vi "探头模板-12.vi"() -> ()   [LabVIEW 2017]
uses:
  <vilib>/Utility/miscctls.llb/LVPoint32TypeDef.ctl
  <vilib>/Utility/miscctls.llb/LVPositionTypeDef.ctl
panel:
  in  "鼠标坐标":T1 caption="坐标"
  out "计算时间":dbl
  in  "坐标映射信号":bool=TRUE
  in  "停止":bool=TRUE
  out "探头地址":T2(ring)
  out "探头状态":T3(ring)=enum."离线"
  out "探头信息":string
  out "测量值":dbl format="%.2g"
  out "单位":enum16{"μ", "m"}(ring)
  out "限值1":string="一级限值："
  out "限值2":string="二级限值："
  out "累积剂量":string="二级限值："
  in  "数据簇":T4
  out "数值":string
  in  "XY图":cluster{timestamp[], dbl[]}[](graph)
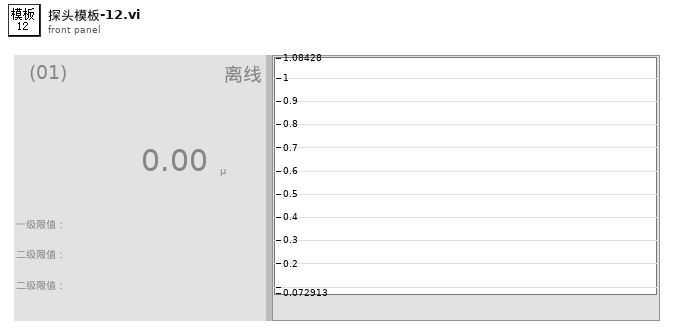
[diagram p1: front panel]
types:
  T1 = typedef "LVPoint32TypeDef.ctl" = cluster{"Horizontal":i32, "Vertical":i32}
  T2 = enum16{"(01)", "(02)", "(03)", "(04)", "(05)", "(06)", "(07)", "(08)", "(09)", "(10)", "(11)", "(12)", "(13)", "(14)", "(15)", "(16)", "(17)", "(18)", "(19)", "(20)", "(21)", "(22)", "(23)", "(24)", "(25)", "(26)", "(27)", "(28)", "(29)", "(30)", "(31)", "(32)", "(33)", "(34)", "(35)"}
  T3 = enum16{"正常", "未启用", "离线", "一级报警", "二级报警", "累积报警"}
  T4 = cluster{"启用状态？":bool, "测量值":cluster{"X":timestamp, "Y":dbl}, "限值簇":cluster{"限值1":dbl, "限值2":dbl, "探头限值":enum16{"一级限值", "二级限值"}}, "报警状态":enum16{"正常", "一级报警", "二级报警", "累积报警"}, "探头信息":string, "探头地址":i32, "累积剂量":cluster{"设备名称":string, "启用累积？":bool, "起始时间":timestamp, "累积剂量":dbl, "累积报警阈值":dbl}}
  T5 = typedef "LVPositionTypeDef.ctl" = cluster{"Left":i32, "Top":i32}
  T6 = cluster{"限值1":dbl, "限值2":dbl, "探头限值":enum16{"一级限值", "二级限值"}}
  T7 = cluster{"设备名称":string, "启用累积？":bool, "起始时间":timestamp, "累积剂量":dbl, "累积报警阈值":dbl}
  T8 = typedef "LVBoundsTypeDef.ctl" = cluster{"Width":u32, "Height":u32}
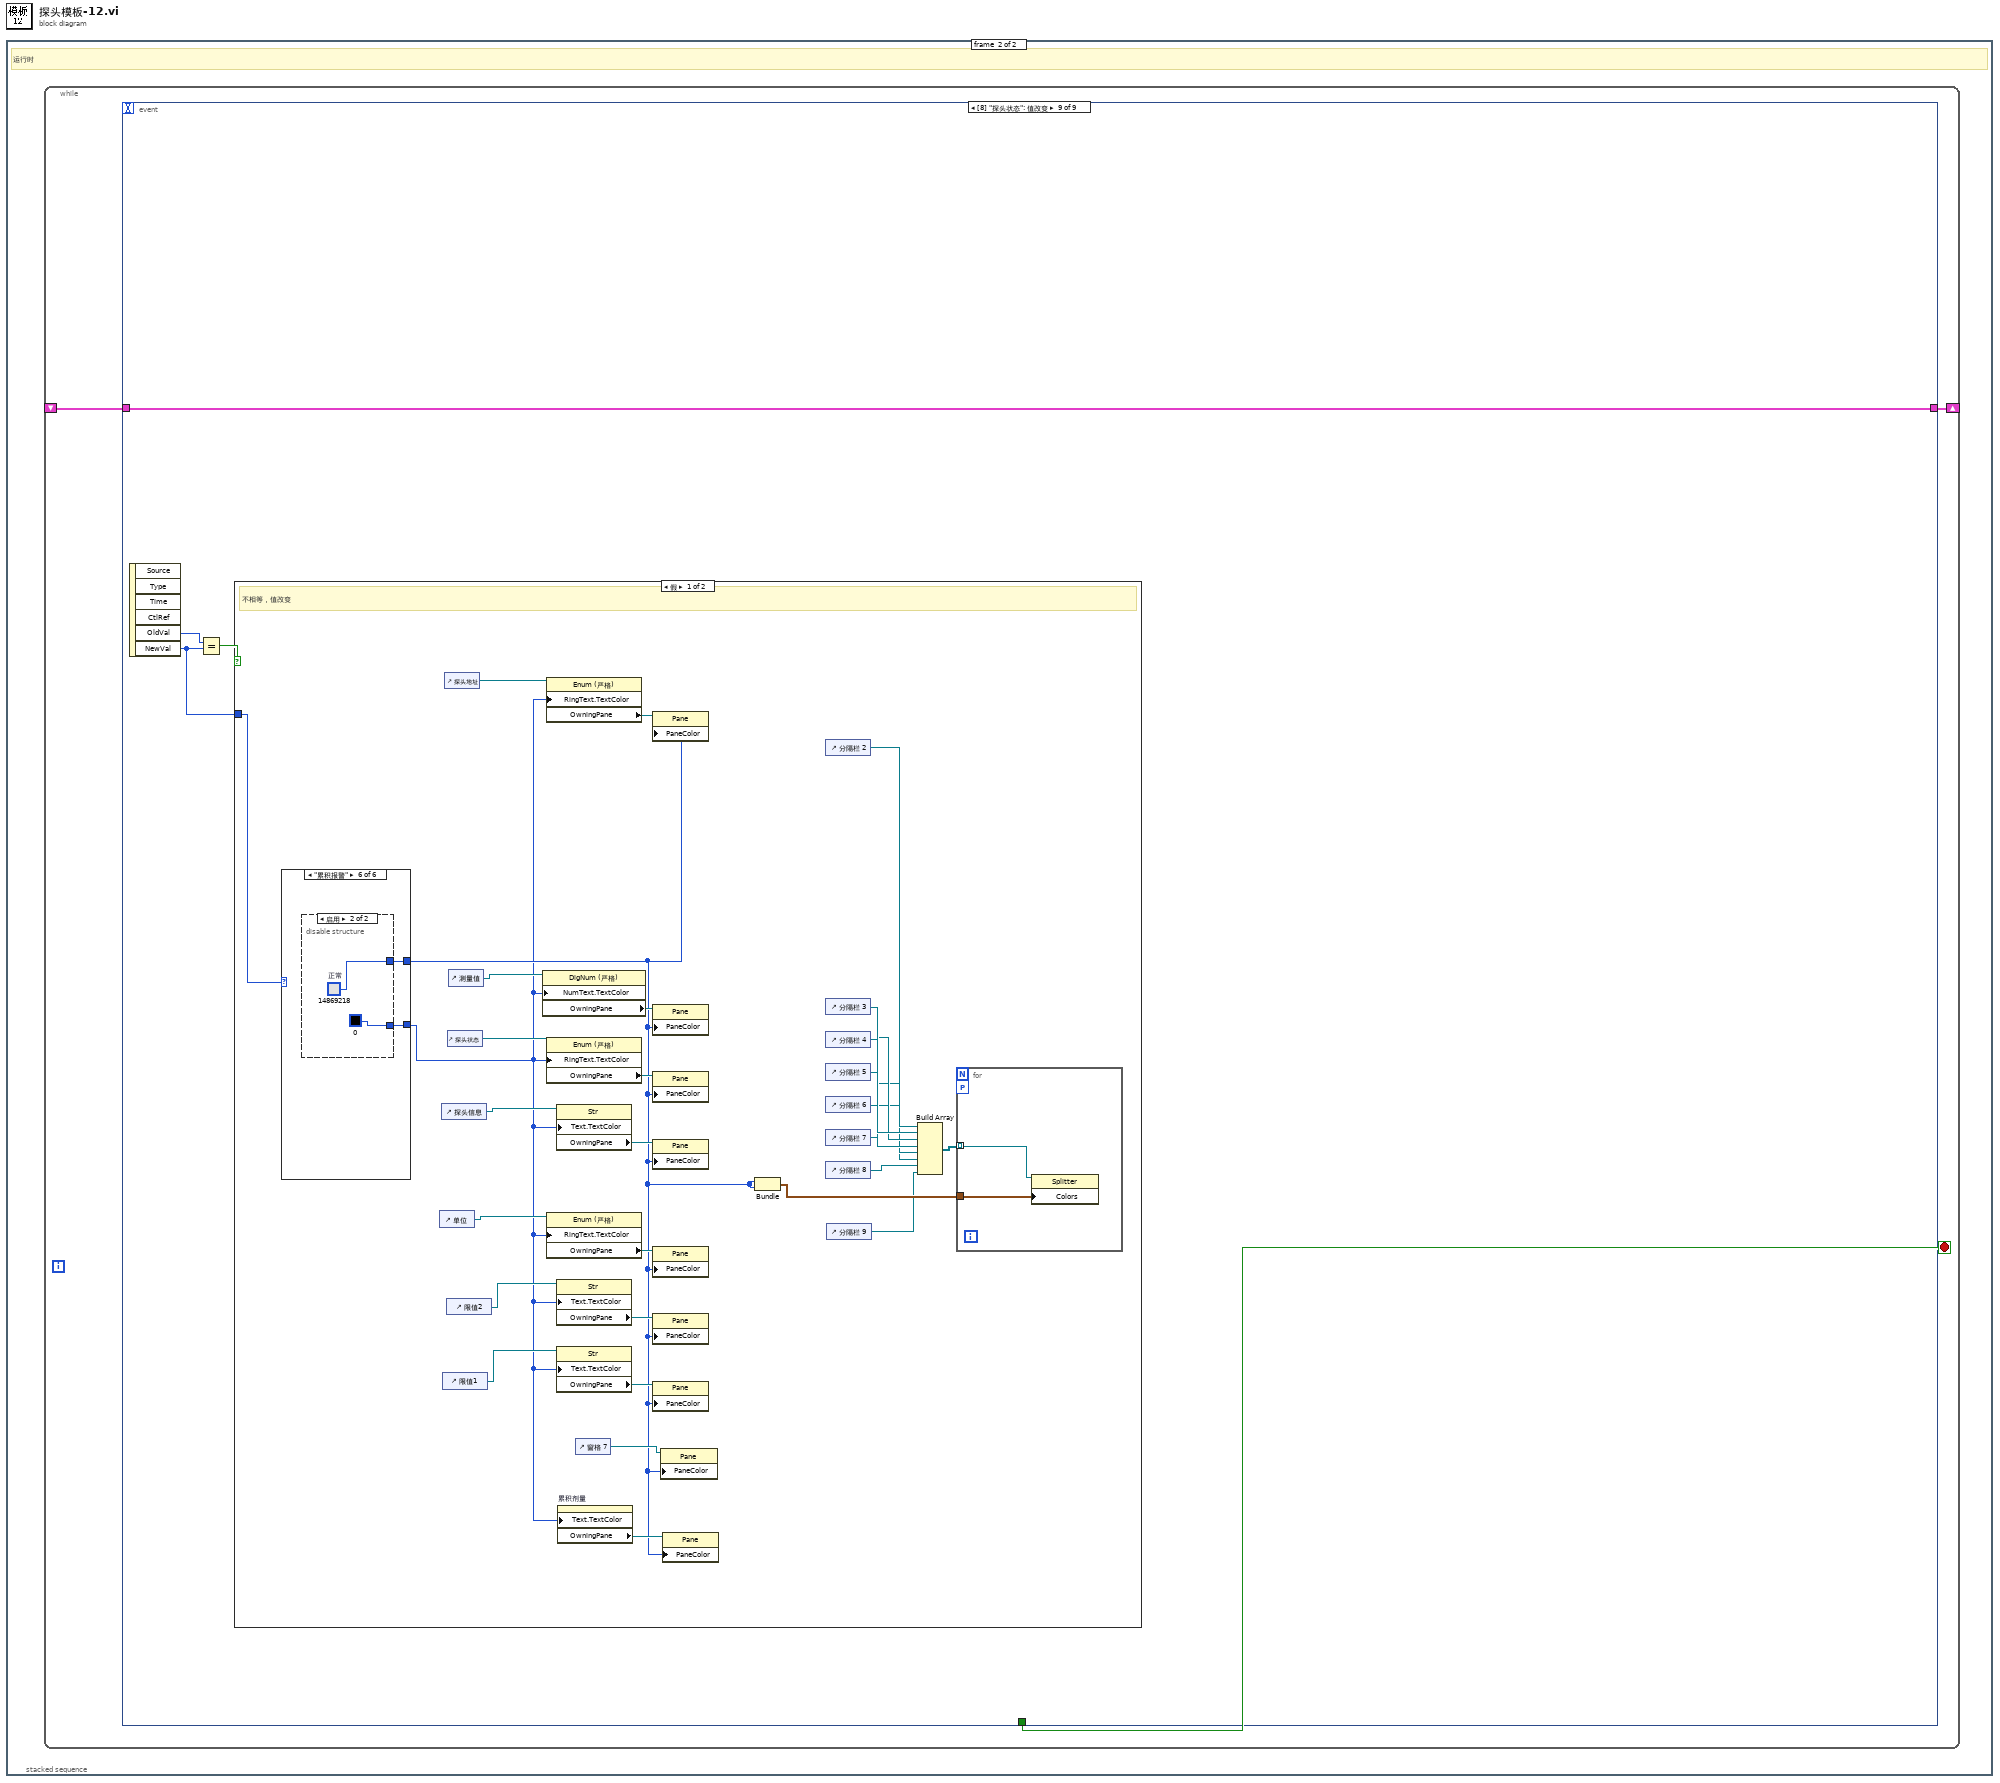
[diagram p0: block diagram]
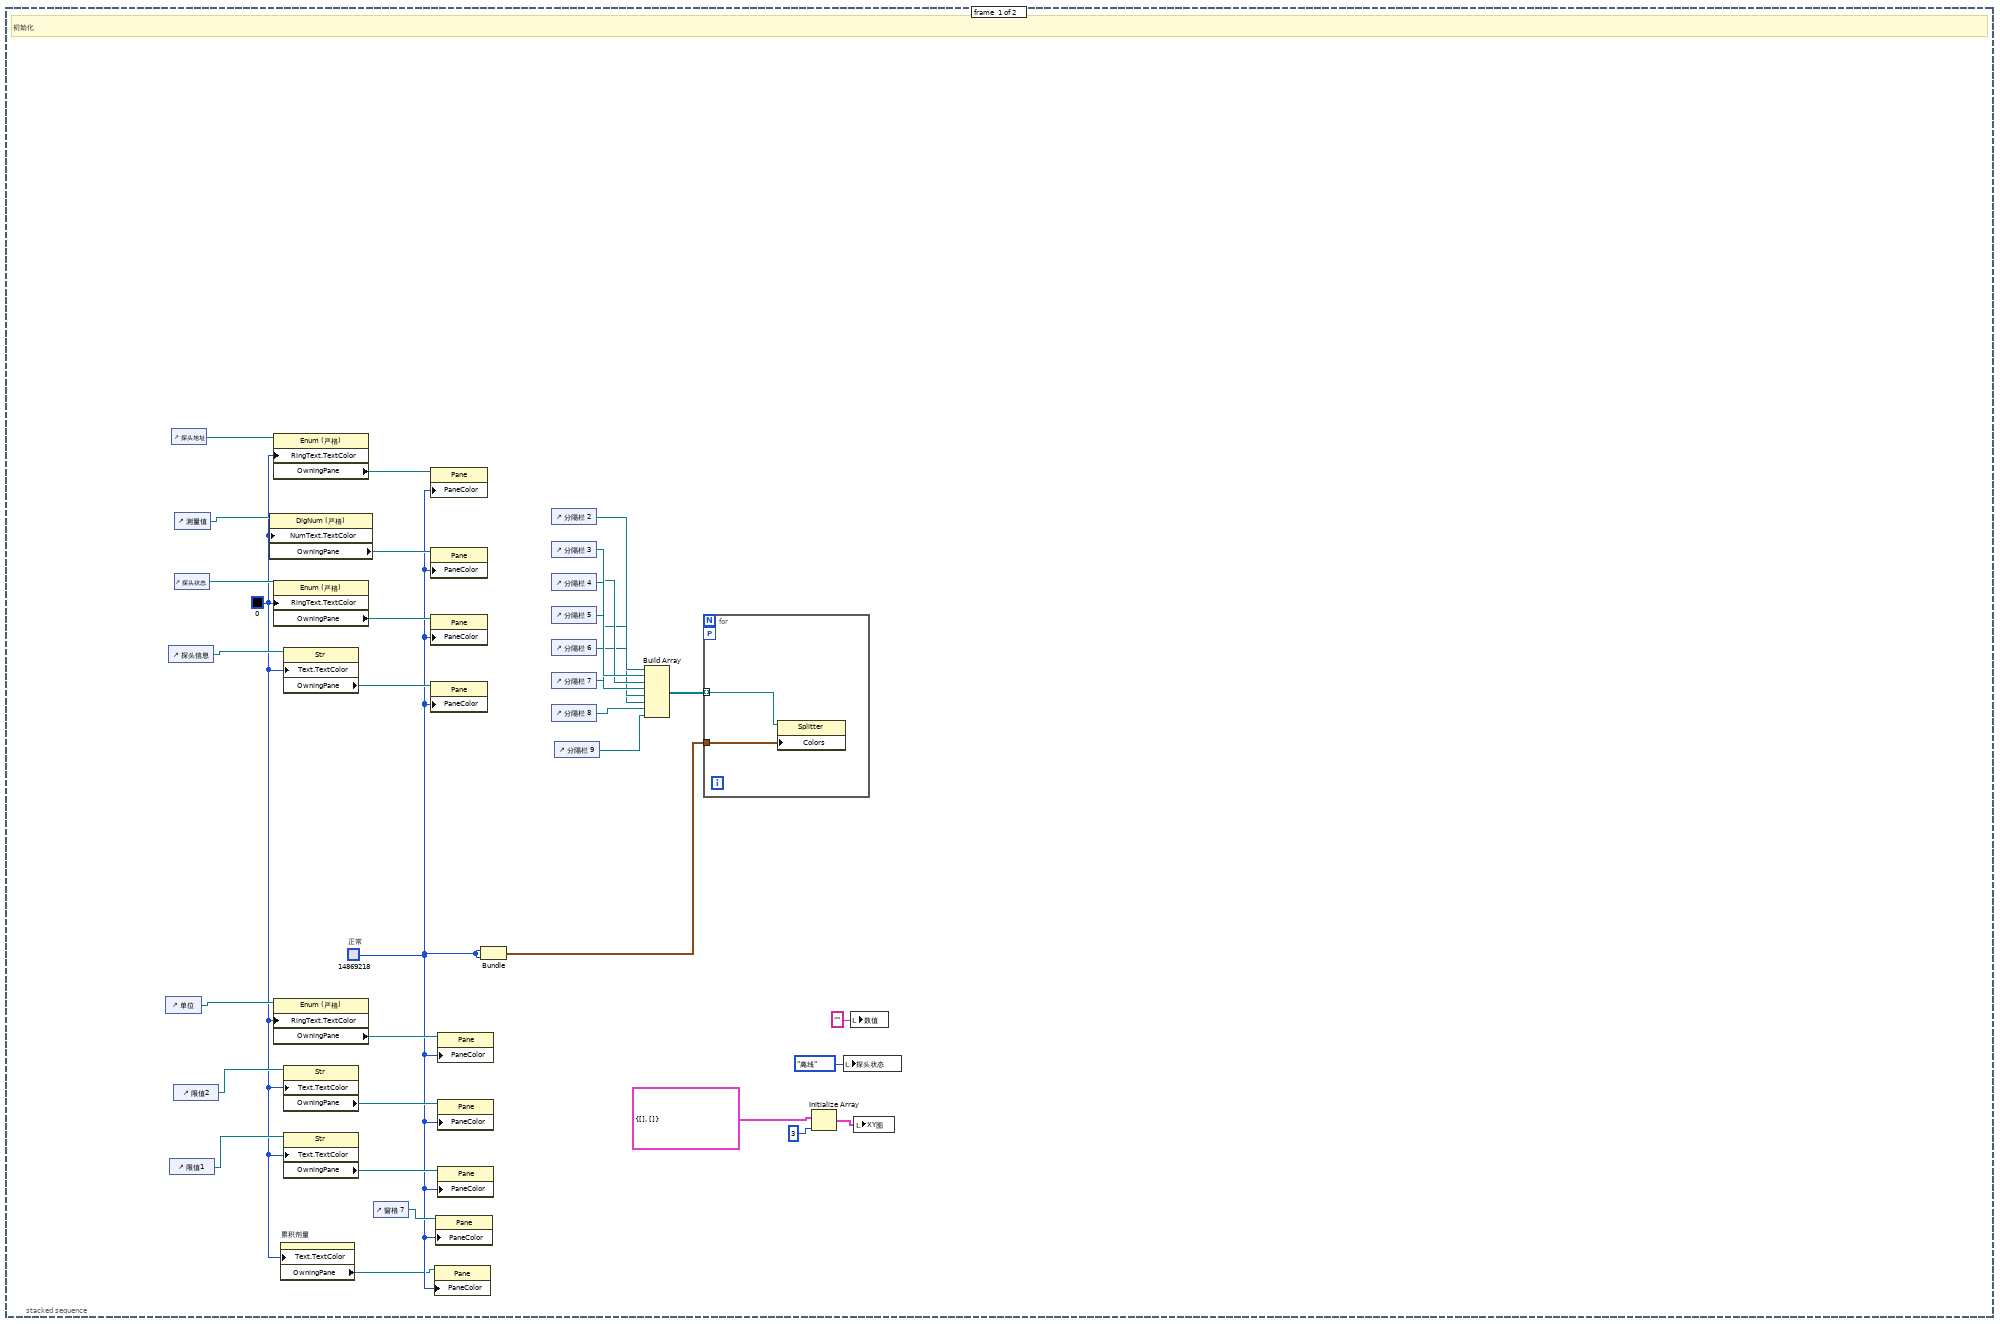
[diagram p2: hidden frame]
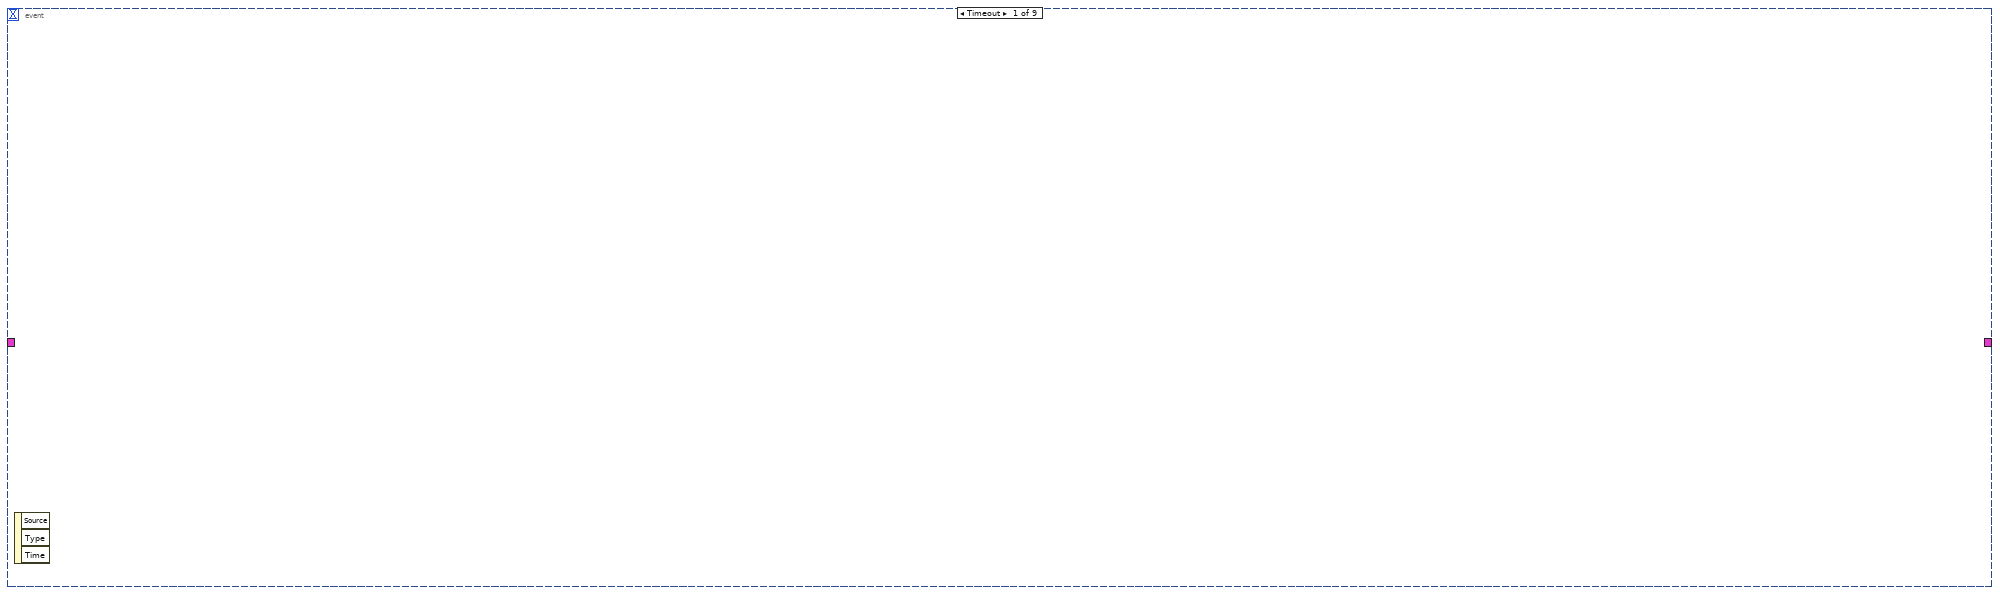
[diagram p3: hidden frame]
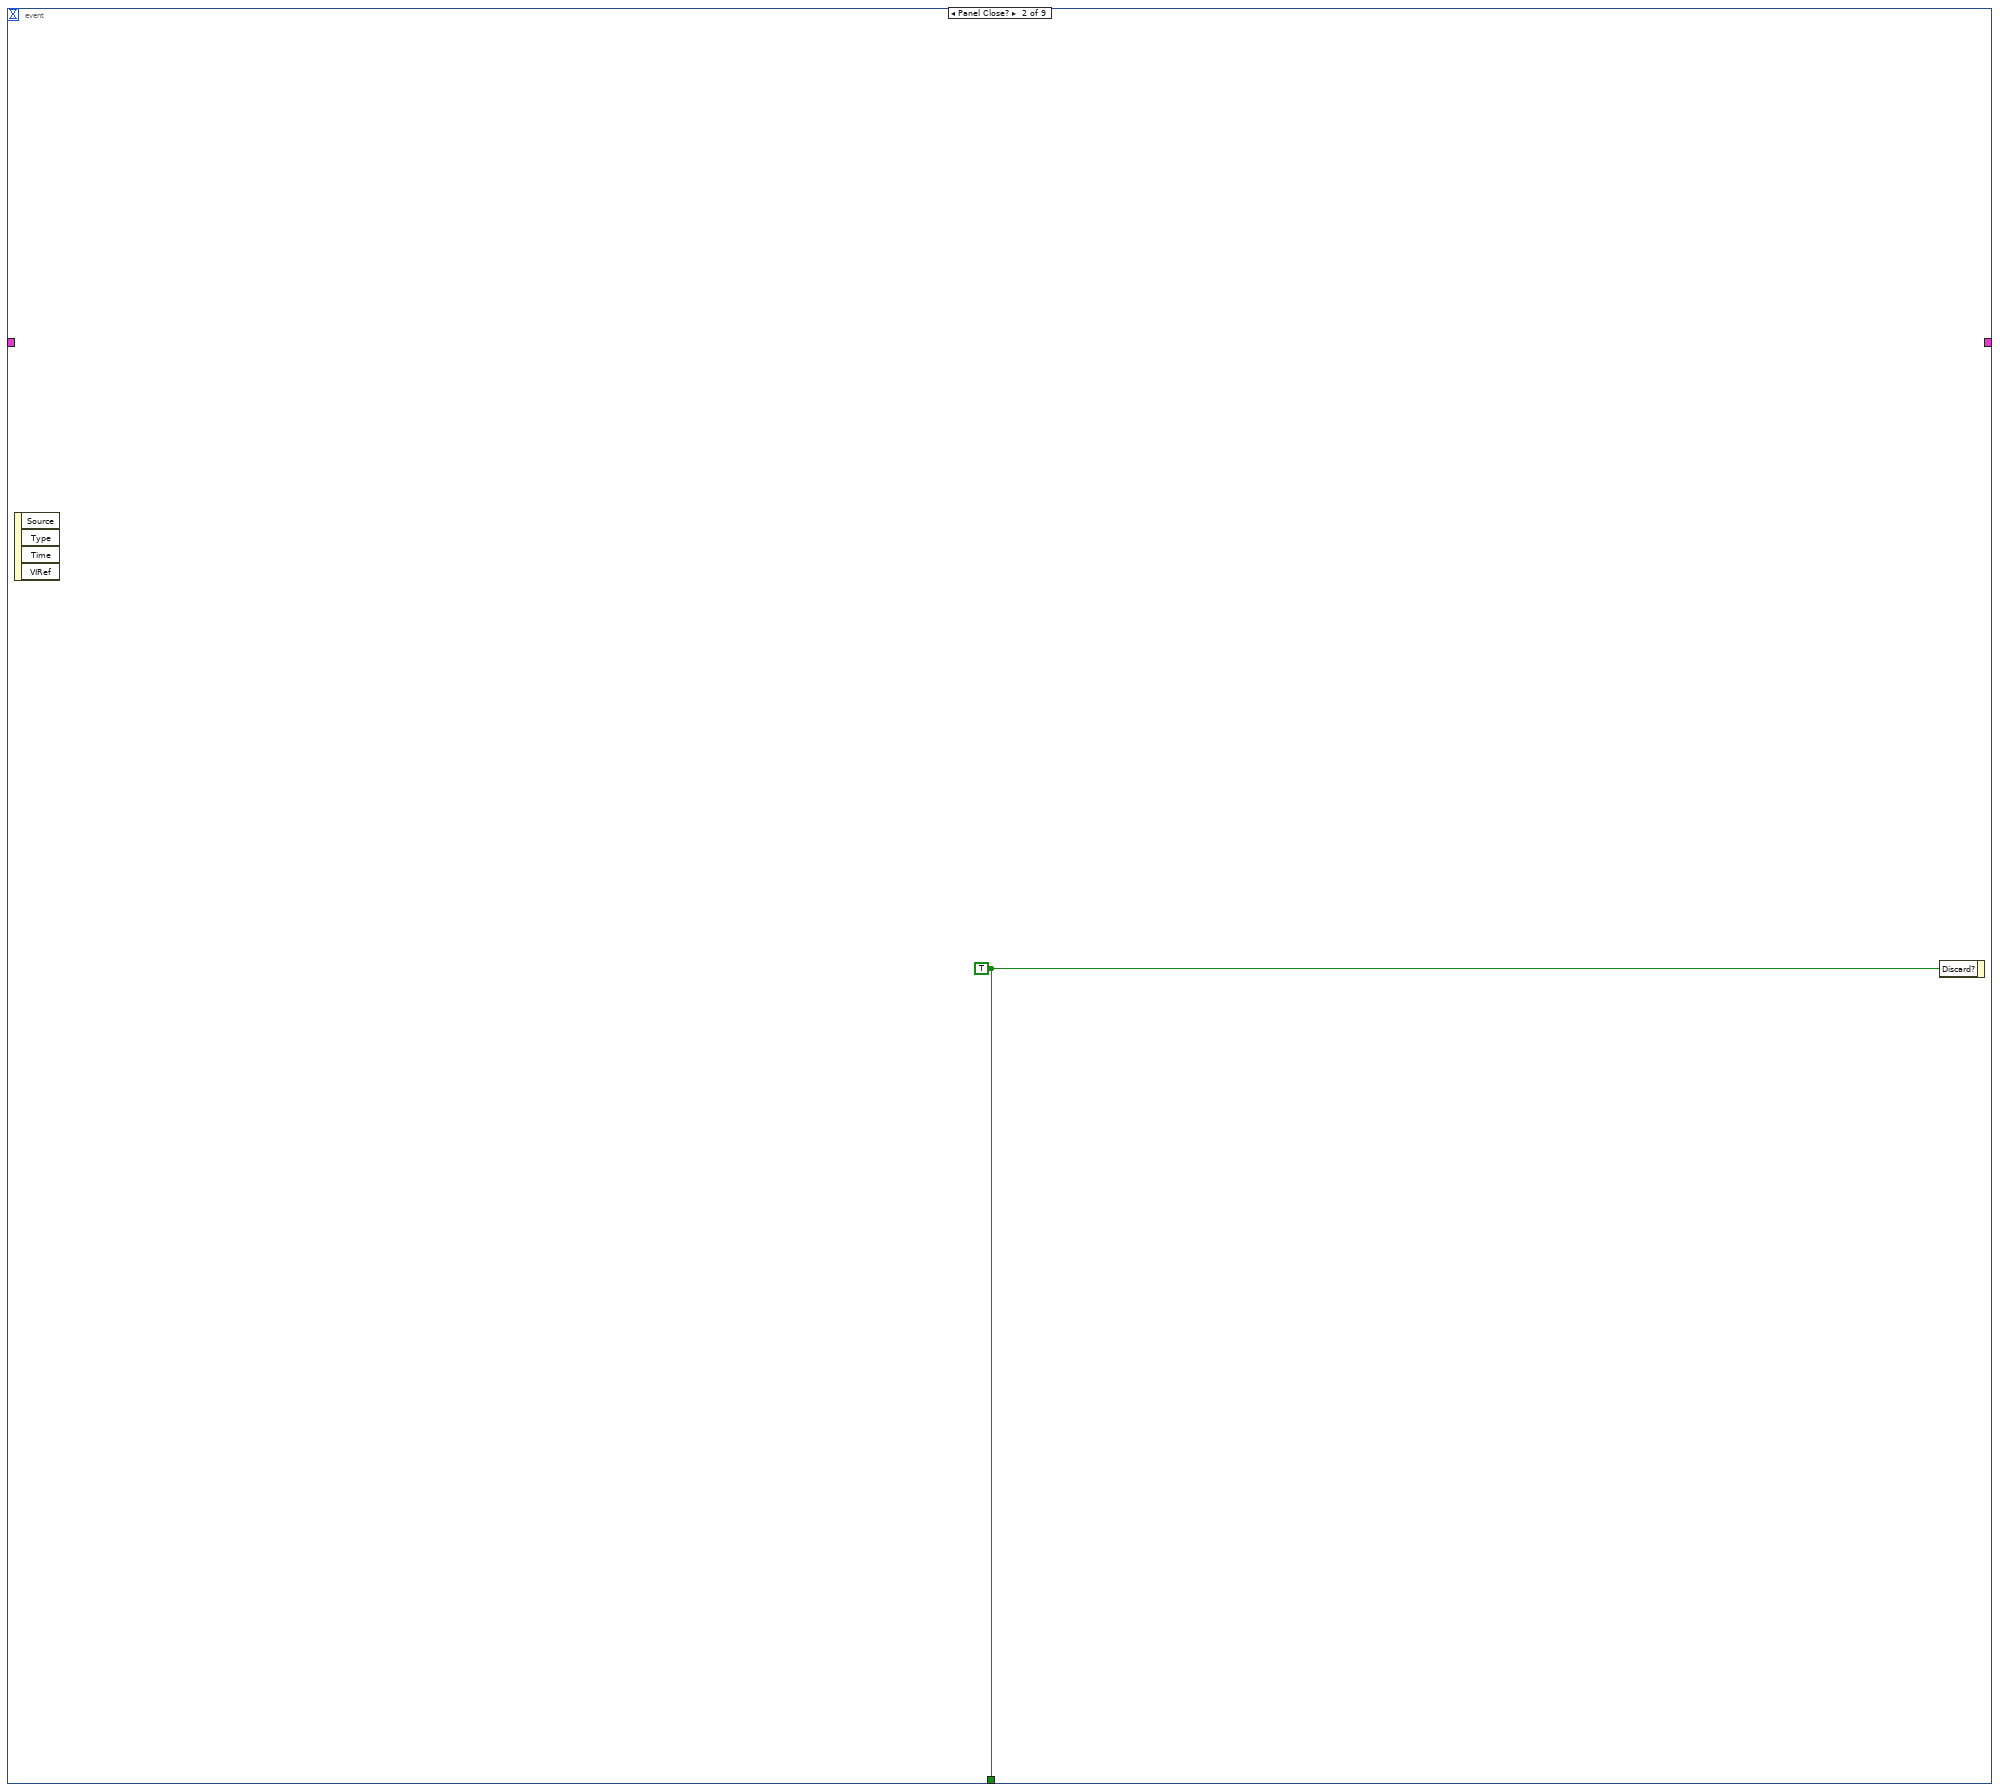
[diagram p4: hidden frame]
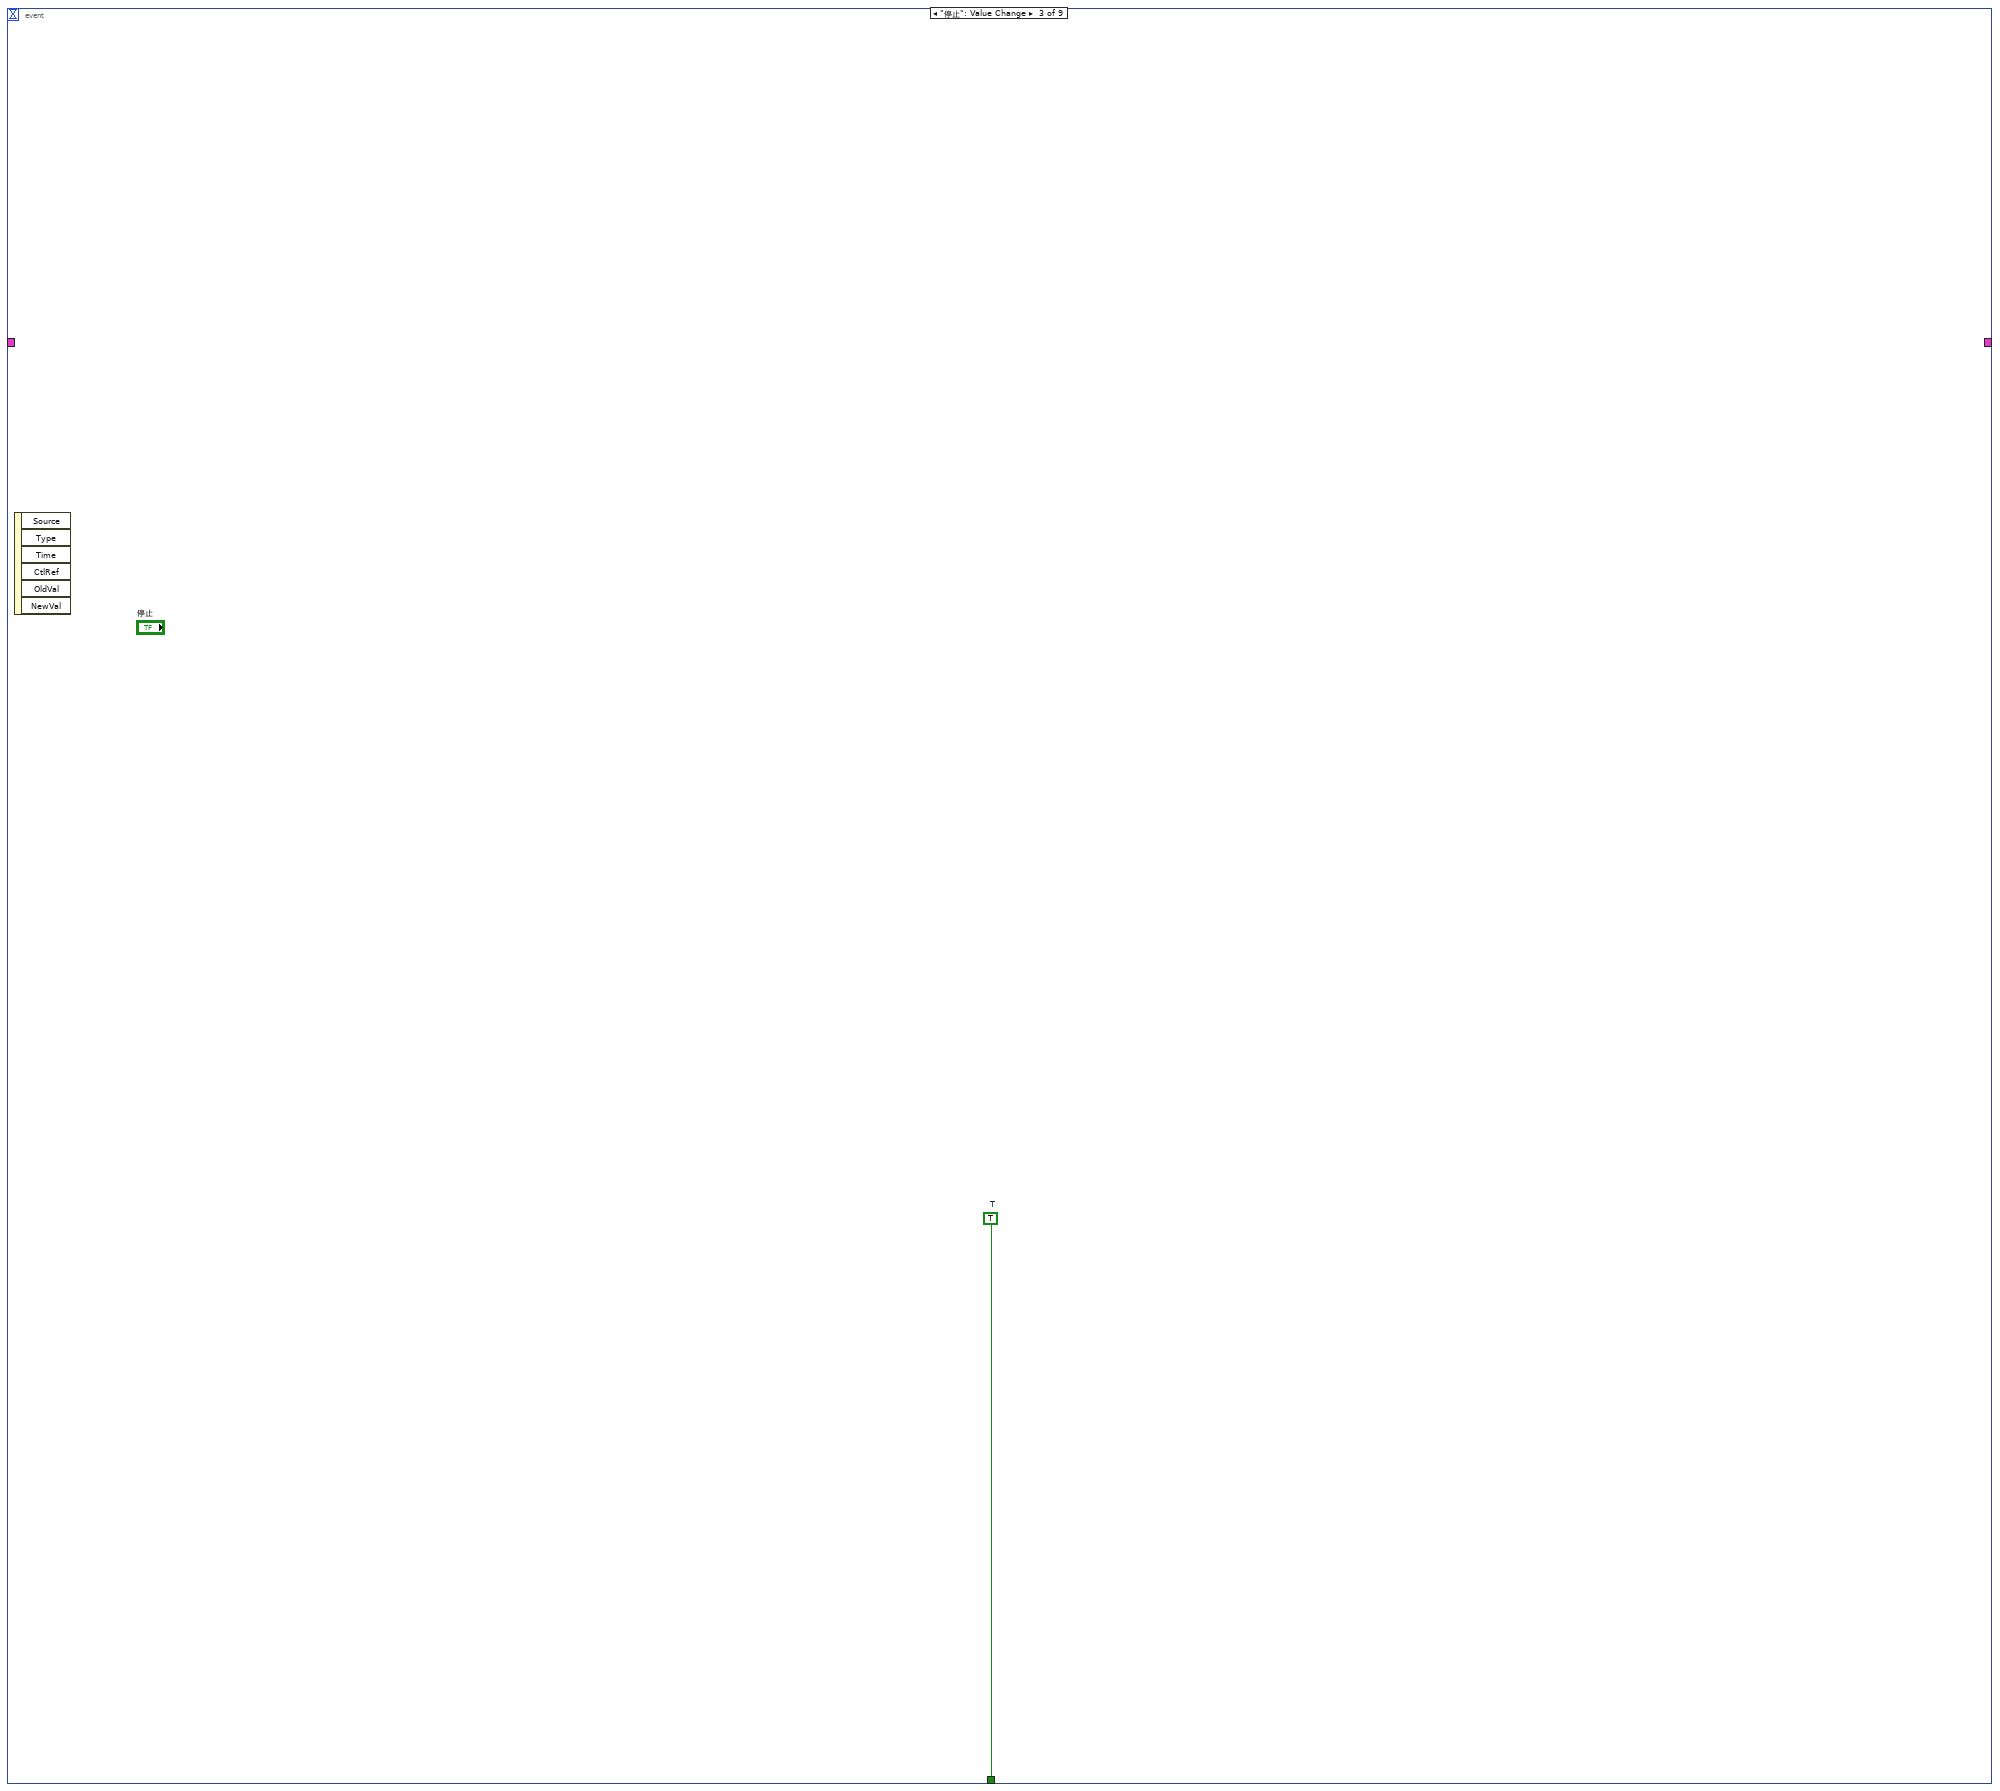
[diagram p5: hidden frame]
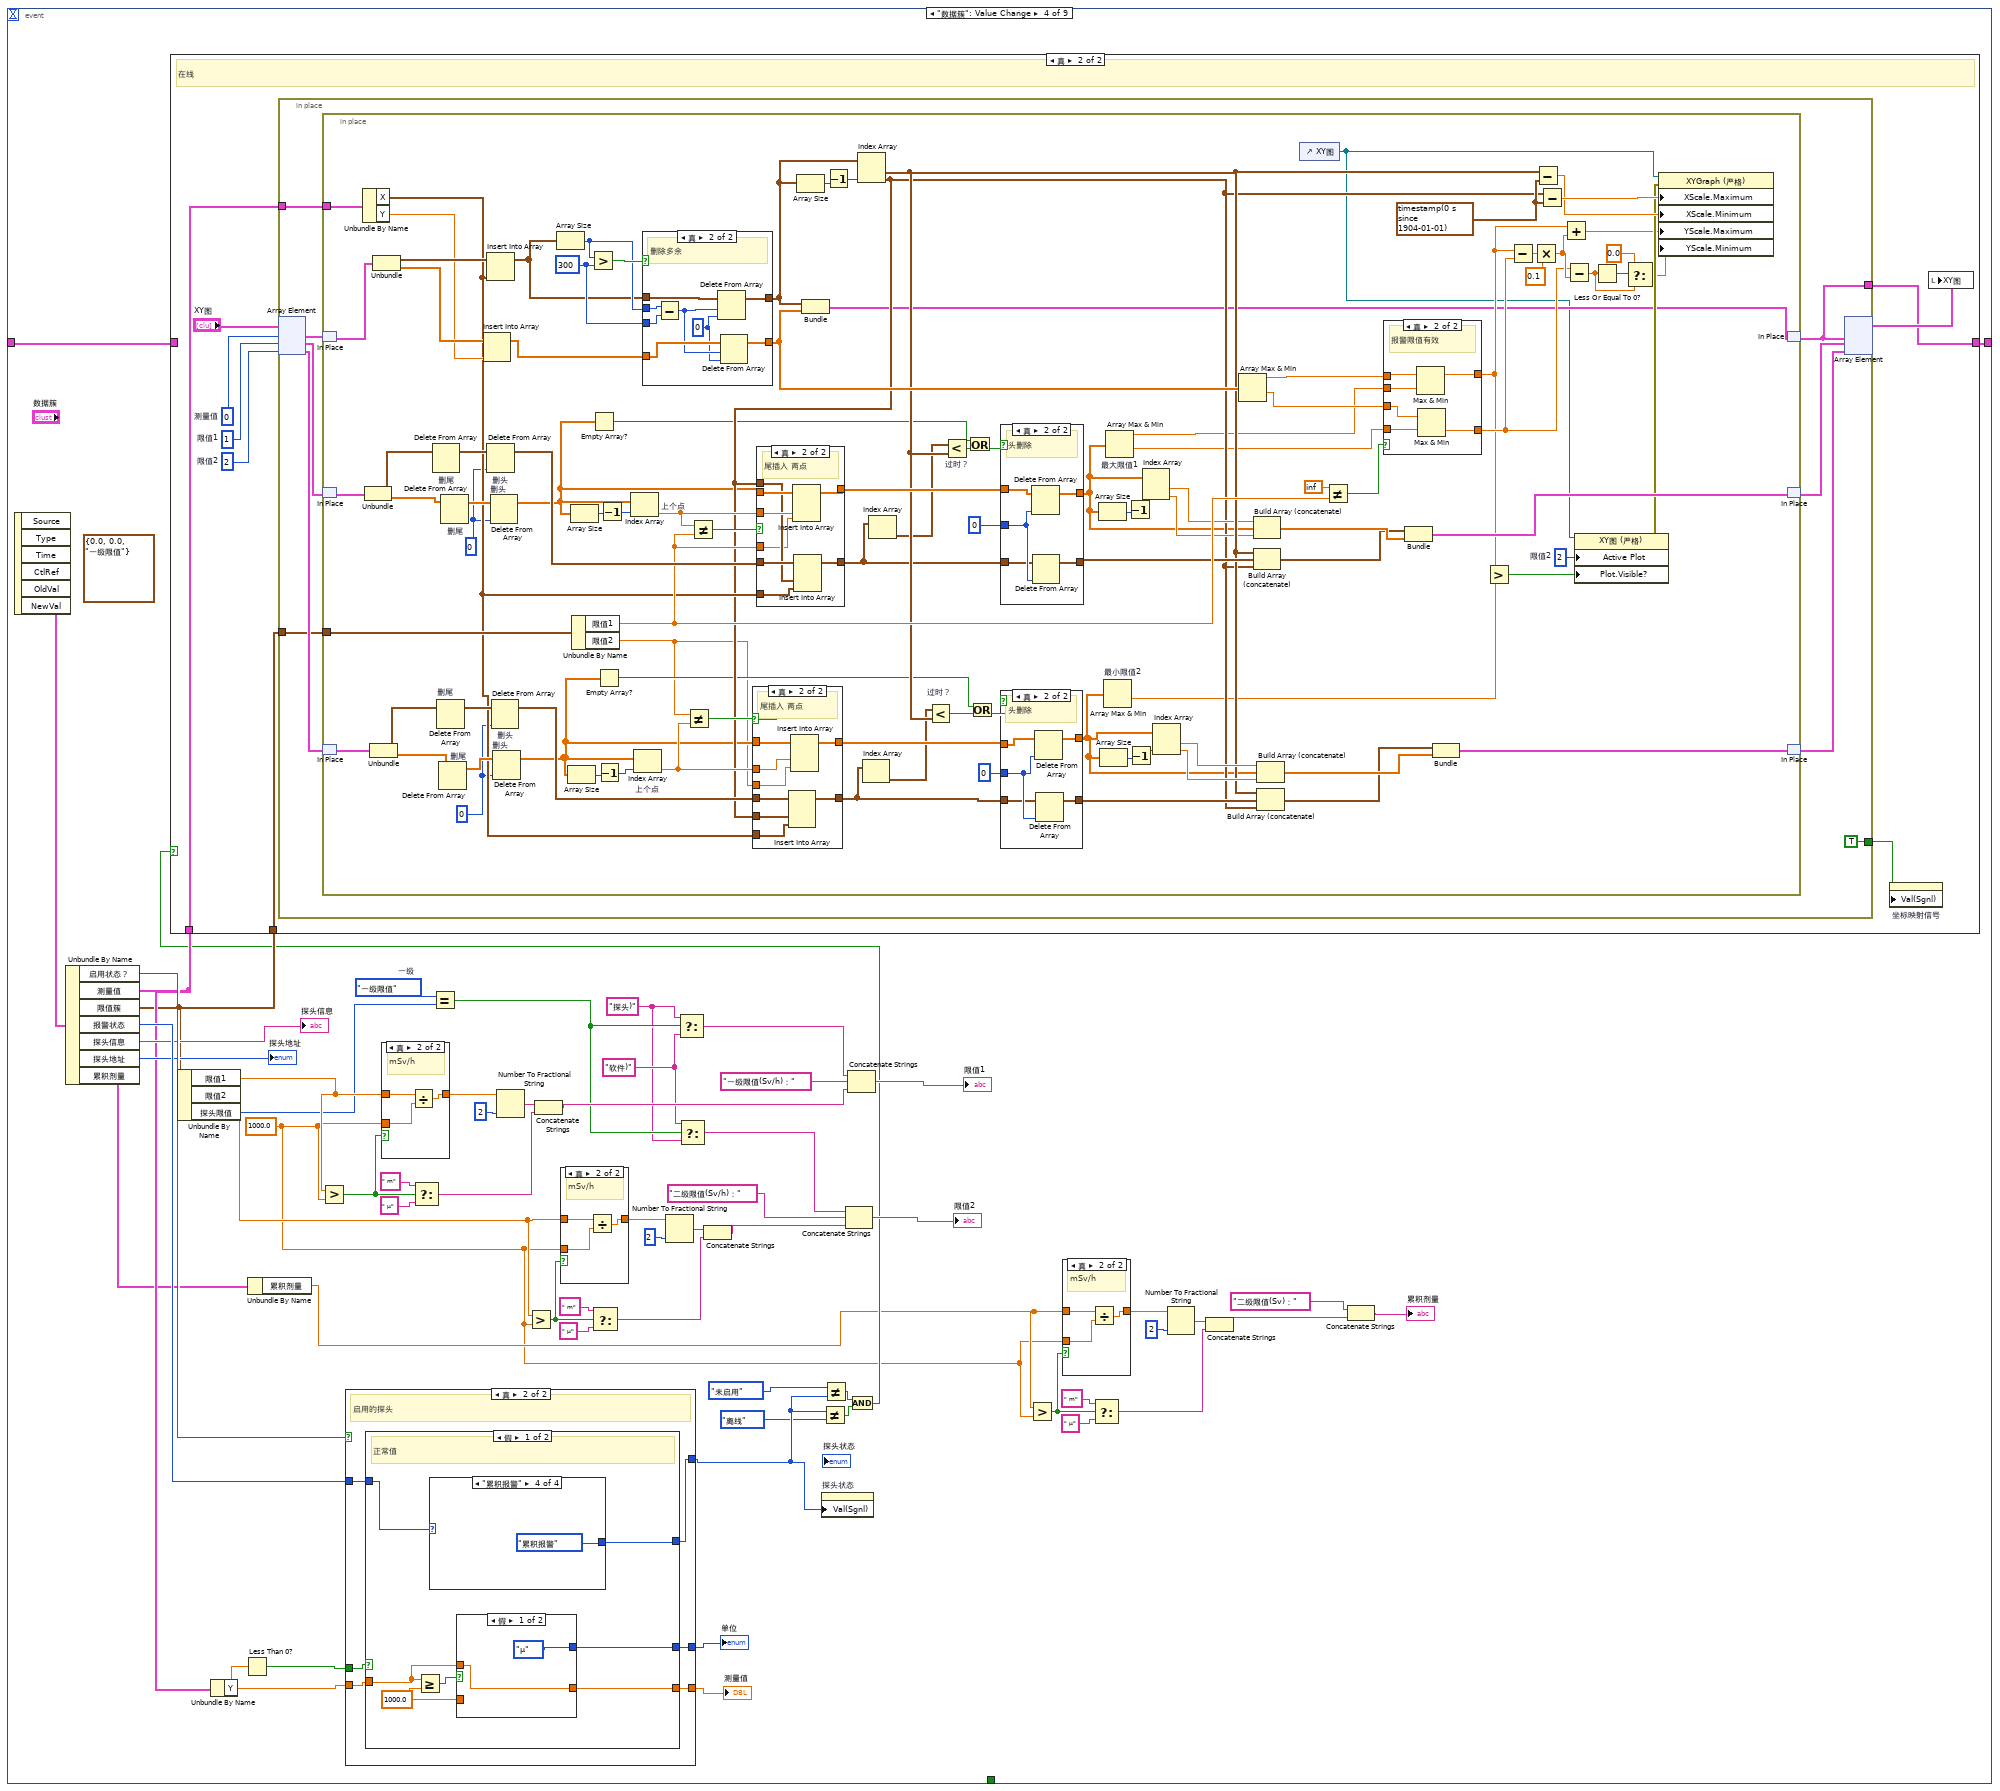
[diagram p6: hidden frame]
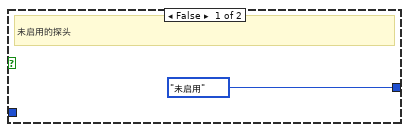
[diagram p15: hidden frame]
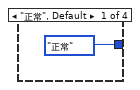
[diagram p16: hidden frame]
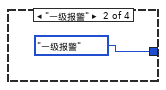
[diagram p17: hidden frame]
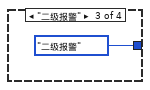
[diagram p18: hidden frame]
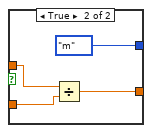
[diagram p19: hidden frame]
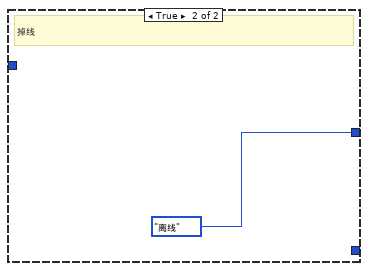
[diagram p20: hidden frame]
diagram:
  n1 = stacked-sequence {
    frame #0 {
      w1 = u32 0
      w3 = u32 14869218  # 正常
      # "初始化"
      n2 = control-ref of="单位"() -> (w22:refnum<vi>)
      n3 = control-ref of="探头信息"() -> (w23:refnum<vi>)
      n4 = control-ref of="限值1"() -> (w20:refnum<vi>)
      n5 = control-ref of="探头地址"() -> (w26:refnum<vi>)
      n6 = control-ref of="限值2"() -> (w21:refnum<vi>)
      n7 = control-ref of="探头状态"() -> (w24:refnum<vi>)
      n8 = control-ref of="测量值"() -> (w25:refnum<vi>)
      n9 = property on="属性节点" class="DigNum (严格)"(reference=w25, "NumText.TextColor"=w1) -> ("OwningPane"=w28:refnum<vi>)  [unwired: 1 in, 2 out]
      n10 = property on="属性节点" class="Enum (严格)"(reference=w26, "RingText.TextColor"=w1) -> ("OwningPane"=w27:refnum<vi>)  [unwired: 1 in, 2 out]
      n11 = property on="属性节点" class="Enum (严格)"(reference=w24, "RingText.TextColor"=w1) -> ("OwningPane"=w29:refnum<vi>)  [unwired: 1 in, 2 out]
      n12 = property on="属性节点" class="Enum (严格)"(reference=w22, "RingText.TextColor"=w1) -> ("OwningPane"=w31:refnum<vi>)  [unwired: 1 in, 2 out]
      n13 = property on="累积剂量" class="Str"("Text.TextColor"=w1) -> ("OwningPane"=w2:refnum<vi>)  [unwired: 2 in, 2 out]
      n14 = property on="属性节点" class="Str"(reference=w23, "Text.TextColor"=w1) -> ("OwningPane"=w30:refnum<vi>)  [unwired: 1 in, 2 out]
      n15 = property on="属性节点" class="Str"(reference=w21, "Text.TextColor"=w1) -> ("OwningPane"=w32:refnum<vi>)  [unwired: 1 in, 2 out]
      n16 = property on="属性节点" class="Str"(reference=w20, "Text.TextColor"=w1) -> ("OwningPane"=w33:refnum<vi>)  [unwired: 1 in, 2 out]
      n17 = control-ref of="窗格 7"() -> (w6:refnum<vi>)
      n18 = property class="Pane"(reference=w27, "PaneColor"=w3) -> ()  [unwired: 1 in, 2 out]
      n19 = property class="Pane"(reference=w28, "PaneColor"=w3) -> ()  [unwired: 1 in, 2 out]
      n20 = property class="Pane"(reference=w29, "PaneColor"=w3) -> ()  [unwired: 1 in, 2 out]
      n21 = property class="Pane"(reference=w30, "PaneColor"=w3) -> ()  [unwired: 1 in, 2 out]
      n22 = property class="Pane"(reference=w2, "PaneColor"=w3) -> ()  [unwired: 1 in, 2 out]
      n23 = property class="Pane"(reference=w6, "PaneColor"=w3) -> ()  [unwired: 1 in, 2 out]
      n24 = property class="Pane"(reference=w31, "PaneColor"=w3) -> ()  [unwired: 1 in, 2 out]
      n25 = property class="Pane"(reference=w32, "PaneColor"=w3) -> ()  [unwired: 1 in, 2 out]
      n26 = property class="Pane"(reference=w33, "PaneColor"=w3) -> ()  [unwired: 1 in, 2 out]
      n27 = Bundle("正常"=w3, "正常"=w3) -> (w12:cluster{"正常":u32, "正常":u32})  [unwired: 1 in]
      n28 = control-ref of="分隔栏 2"() -> (w19:refnum<vi>)
      n29 = control-ref of="分隔栏 3"() -> (w18:refnum<vi>)
      n30 = control-ref of="分隔栏 4"() -> (w17:refnum<vi>)
      n31 = control-ref of="分隔栏 5"() -> (w16:refnum<vi>)
      n32 = control-ref of="分隔栏 6"() -> (w15:refnum<vi>)
      n33 = control-ref of="分隔栏 7"() -> (w14:refnum<vi>)
      n34 = control-ref of="分隔栏 8"() -> (w13:refnum<vi>)
      n35 = control-ref of="分隔栏 9"() -> (w4:refnum<vi>)
      n36 = Build Array(w19, w18, w17, w16, w15, w14, w13, w4) -> (w11:refnum<vi>[])
      n37 = for {
        tunnel: w12 -> [w35]
        workers-P: _ -> [_]
        tunnel: w11 -> [w34] mode=indexing
        n38 = property on="属性节点" class="Splitter"(reference=w34, "Colors"=w35) -> ()  [unwired: 1 in, 2 out]
      }
      n39 = Initialize Array(cluster{timestamp[], dbl[]} {[], []}, 3 ("维数大小")) -> (w7:cluster{timestamp[], dbl[]}[])
      n40 = local write "探头状态"(enum16{"正常", "未启用", "离线", "一级报警", "二级报警"}."离线" ("探头状态")) -> ()
      n41 = local write "数值"("" ("数值")) -> ()
      n42 = local write "XY图"(w7) -> ()
    }
    frame #1 {
      # "运行时"
      n43 = while {
        shift-right: [w37] -> _
        shift-left: _ -> [w36]
        stop <- w38 stop-if-true
        n44 = event shown="[8] \"探头状态\": 值改变" {
          selector: _ -> [_ _ _ _ _ _ _ _ _]
          dyn-events: _ -> [_ _ _ _ _ _ _ _ _]
          timeout: _ -> [_ _ _ _ _ _ _ _ _]
          tunnel: [_ w39 w40 _ _ _ _ _ _] -> w38
          tunnel: [_ _ _ w68 w311 w365 w367 w369 w372] -> w37
          tunnel: w36 -> [_ _ _ w61 w311 w365 w367 w369 w372]
          event Timeout {
            n45 = event-data() -> ()  [unwired: 1 in, 3 out]
          }
          event Panel Close? {
            w39 = TRUE ("放弃？")
            n46 = event-data() -> ()  [unwired: 1 in, 4 out]
            n47 = event-data("Discard?"=w39) -> ()  [unwired: 1 in, 1 out]
          }
          event "停止": Value Change {
            w40 = TRUE  # T
            n48 = event-data() -> ()  [unwired: 1 in, 6 out]
          }
          event "数据簇": Value Change {
            w46 = enum16{"一级限值", "二级限值"}."一级限值"  # 一级
            w44 = "软件)" ("字符串")
            w43 = "探头)" ("字符串")
            (unwired) T6 {"限值1"=0.0, "限值2"=0.0, "探头限值"=enum."一级限值"} ("探头限值簇")
            w49 = 1000.0 ("y")
            n49 = event-data() -> ("NewVal"=w101:T4)  [unwired: 1 in, 5 out]
            n50 = Unbundle By Name(w101) -> ("启用状态？"=w78:bool, "测量值"=w70:cluster{"X":timestamp, "Y":dbl}, "限值簇"=w69:T6, "报警状态"=w77:enum16{"正常", "一级报警", "二级报警", "累积报警"}, "探头信息"=→"探头信息":string, "探头地址"=→"探头地址":i32, "累积剂量"=w60:T7)
            n51 = Unbundle By Name(w69) -> ("限值1"=w97:dbl, "限值2"=w99:dbl, "探头限值"=w47:enum16{"一级限值", "二级限值"})
            n52 = Unbundle By Name(w70) -> ("Y"=w80:dbl)
            n53 = Less Than 0?(x=w80) -> (x < 0?=w79:bool)
            n54 = Unbundle By Name(w60) -> ("累积剂量"=w50:dbl)
            n55 = Greater?(x=w97, y=w49) -> (0:w84:bool)
            n56 = case shown="真" w78 {
              tunnel: w79 -> [_ w284]
              tunnel: w80 -> [_ w283]
              tunnel: [_ w282] -> w73
              tunnel: [_ w281] -> w74
              tunnel: [enum16{"正常", "未启用", "离线", "一级报警", "二级报警"}."未启用" ("探头状态") w280] -> w65
              tunnel: w77 -> [_ w279]
              frame False {
                # "未启用的探头"
              }
              frame True {
                # "启用的探头"
                n57 = case shown="假" w284 {
                  tunnel: w283 -> [w290 _]
                  tunnel: [w288 _] -> w282
                  tunnel: [w287 _] -> w281
                  tunnel: [w285 enum16{"正常", "未启用", "离线", "一级报警", "二级报警"}."离线" ("探头状态")] -> w280
                  tunnel: w279 -> [w286 _]
                  frame False {
                    w289 = 1000.0 ("y")
                    # "正常值"
                    n58 = Greater Or Equal?(x=w290, y=w289) -> (x >= y?=w291:bool)
                    n59 = case shown="\"累积报警\"" w286 {
                      tunnel: [enum16{"正常", "未启用", "离线", "一级报警", "二级报警"}."正常" ("探头状态") enum16{"正常", "未启用", "离线", "一级报警", "二级报警"}."一级报警" ("探头状态") enum16{"正常", "未启用", "离线", "一级报警", "二级报警"}."二级报警" ("探头状态") T3."累积报警" ("探头状态")] -> w285
                      frame "正常", Default {
                      }
                      frame "一级报警" {
                      }
                      frame "二级报警" {
                      }
                      frame "累积报警" {
                      }
                    }
                    n60 = case shown="假" w291 {
                      tunnel: w290 -> [w297 w301]
                      tunnel: w289 -> [_ w300]
                      tunnel: [w297 w299] -> w288
                      tunnel: [enum16{"μ", "m"}."μ" ("单位") enum16{"μ", "m"}."m" ("单位")] -> w287
                      frame False {
                      }
                      frame True {
                        n61 = Divide(x=w301, y=w300) -> (x/y=w299:dbl)
                      }
                    }
                  }
                  frame True {
                    # "掉线"
                  }
                }
              }
            }
            "测量值" <- w73
            "单位" <- w74
            n62 = case shown="真" w84 {
              tunnel: w97 -> [w307 w310]
              tunnel: w49 -> [_ w309]
              tunnel: [w307 w308] -> w89
              frame False {
                # "uSv/h"
              }
              frame True {
                # "mSv/h"
                n63 = Divide(x=w310, y=w309) -> (x/y=w308:dbl)
              }
            }
            n64 = Select(t=" m" ("F-格式字符串"), s=w84, f=" μ" ("F-格式字符串")) -> (s? t:f=w88:string)
            n65 = Equal?(x=w46, y=w47) -> (x = y?=w45:bool)
            n66 = Number To Fractional String(number=w89, precision (6)=i16 2 ("精度(6)")) -> (F-format string=w85:string)  [unwired: 2 in]
            n67 = Greater?(x=w99, y=w49) -> (0:w91:bool)
            n68 = Concatenate Strings(w85, w88) -> (w98:string)
            n69 = case shown="真" w91 {
              tunnel: w99 -> [w303 w306]
              tunnel: w49 -> [_ w305]
              tunnel: [w303 w304] -> w96
              frame False {
                # "uSv/h"
              }
              frame True {
                # "mSv/h"
                n70 = Divide(x=w306, y=w305) -> (x/y=w304:dbl)
              }
            }
            n71 = Select(t=" m" ("F-格式字符串"), s=w91, f=" μ" ("F-格式字符串")) -> (s? t:f=w95:string)
            n72 = Number To Fractional String(number=w96, precision (6)=i16 2 ("精度(6)")) -> (F-format string=w92:string)  [unwired: 2 in]
            n73 = Select(t=w43, s=w45, f=w44) -> (s? t:f=w42:string)
            n74 = Select(t=w44, s=w45, f=w43) -> (s? t:f=w41:string)
            n75 = Concatenate Strings(w92, w95) -> (w100:string)
            n76 = Not Equal?(x=w65, y=enum16{"正常", "未启用", "离线", "一级报警", "二级报警"}."离线" ("探头状态")) -> (x != y?=w66:bool)
            n77 = property on="探头状态" class="Enum (严格)"("Val(Sgnl)"=w65) -> ()  [unwired: 2 in, 2 out]
            n78 = Not Equal?(x=enum16{"正常", "未启用", "离线", "一级报警", "二级报警"}."未启用" ("探头状态"), y=w65) -> (x != y?=w67:bool)
            n79 = Concatenate Strings(w41, "二级限值(Sv/h)：" ("字符串"), w100) -> (→"限值2":string)
            n80 = Concatenate Strings(w42, "一级限值(Sv/h)：" ("字符串"), w98) -> (→"限值1":string)
            n81 = And(x=w67, y=w66) -> (x .and. y?=w62:bool)
            n82 = case shown="真" w62 {
              tunnel: w70 -> [_ w115]
              tunnel: w69 -> [_ w114]
              tunnel: [w106 w108] -> w68
              tunnel: w61 -> [w106 _]
              frame False {
                # "不在线"
              }
              frame True {
                w110 = 2  # 限值2
                w111 = 1  # 限值1
                w112 = 0  # 测量值
                # "在线"
                n83 = in-place {
                  in-place-border: w115 -> [w124]
                  in-place-border: w114 -> [w120]
                  in-place-border: [w117] -> w108
                  in-place-border: [TRUE ("值(信号)")] -> w107
                  n84 = in-place-array #1("XY图", w112, w111, w110) -> (w123:cluster{timestamp[], dbl[]}, w121:cluster{timestamp[], dbl[]}, w122:cluster{timestamp[], dbl[]})
                  n85 = in-place {
                    in-place-border: w124 -> [w219]
                    in-place-border: w120 -> [w213]
                    w149 = 0 ("索引")
                    w150 = 0 ("索引")
                    w211 = u32 2  # 限值2
                    w220 = 300 ("y")
                    w225 = timestamp(0 s since 1904-01-01)
                    n86 = in-place-match #2(w123) -> (w214:cluster{timestamp[], dbl[]})
                    n87 = in-place-match #3(w121) -> (w179:cluster{timestamp[], dbl[]})
                    n88 = in-place-match #4(w122) -> (w160:cluster{timestamp[], dbl[]})
                    n89 = Unbundle By Name(w219) -> ("X"=w159:timestamp, "Y"=w210:dbl)
                    n90 = Unbundle(w179) -> (w183:timestamp[], w182:dbl[])
                    n91 = Unbundle(w160) -> (w164:timestamp[], w163:dbl[])
                    n92 = Unbundle(w214) -> (w218:timestamp[], w217:dbl[])
                    n93 = Delete From Array "删尾"(array=w183) -> (array with subset deleted=w184:timestamp[])  [unwired: 2 in, 1 out]
                    n94 = Delete From Array "删尾"(array=w164) -> (array with subset deleted=w165:timestamp[])  [unwired: 2 in, 1 out]
                    n95 = Delete From Array "删尾"(array=w163) -> (array with subset deleted=w162:dbl[])  [unwired: 2 in, 1 out]
                    n96 = Delete From Array "删尾"(array=w182) -> (array with subset deleted=w181:dbl[])  [unwired: 2 in, 1 out]
                    n97 = Insert Into Array(array=w217, new element=w210) -> (w215:dbl[])  [unwired: 1 in]
                    n98 = Insert Into Array(array=w218, new element=w159) -> (w216:timestamp[])  [unwired: 1 in]
                    n99 = Delete From Array "删头"(array=w184, index=w150) -> (array with subset deleted=w187:timestamp[])  [unwired: 1 in, 1 out]
                    n100 = Delete From Array "删头"(array=w181, index=w150) -> (array with subset deleted=w138:dbl[])  [unwired: 1 in, 1 out]
                    n101 = Delete From Array "删头"(array=w165, index=w149) -> (array with subset deleted=w169:timestamp[])  [unwired: 1 in, 1 out]
                    n102 = Delete From Array "删头"(array=w162, index=w149) -> (array with subset deleted=w137:dbl[])  [unwired: 1 in, 1 out]
                    n103 = Array Size(array=w216) -> (size(s)=w221:i32)
                    n104 = Array Size(array=w137) -> (size(s)=w166:i32)
                    n105 = Array Size(array=w138) -> (size(s)=w180:i32)
                    n106 = Unbundle By Name(w213) -> ("限值1"=w178:dbl, "限值2"=w132:dbl)
                    n107 = Greater?(x=w221, y=w220) -> (0:w222:bool)
                    n108 = Empty Array?(array=w138) -> (empty?=w136:bool)
                    n109 = Empty Array?(array=w137) -> (empty?=w135:bool)
                    n110 = Decrement(x=w166) -> (x-1=w167:i32)
                    n111 = Decrement(x=w180) -> (x-1=w185:i32)
                    n112 = Index Array "上个点"(array=w138, index=w185) -> (element=w148:dbl)
                    n113 = Index Array "上个点"(array=w137, index=w167) -> (element=w147:dbl)
                    n114 = case shown="真" w222 {
                      tunnel: w216 -> [w269 w277]
                      tunnel: w221 -> [_ w276]
                      tunnel: w220 -> [_ w275]
                      tunnel: [w269 w274] -> w209
                      tunnel: w215 -> [w268 w273]
                      tunnel: [w268 w270] -> w205
                      frame False {
                      }
                      frame True {
                        w271 = 0 ("索引")
                        # "删除多余"
                        n115 = Subtract(x=w276, y=w275) -> (x-y=w272:i32)
                        n116 = Delete From Array(array=w277, length=w272, index=w271) -> (array with subset deleted=w274:timestamp[])  [unwired: 1 out]
                        n117 = Delete From Array(array=w273, length=w272, index=w271) -> (array with subset deleted=w270:dbl[])  [unwired: 1 out]
                      }
                    }
                    n118 = Not Equal?(x=w132, y=w147) -> (x != y?=w161:bool)
                    n119 = Not Equal?(x=w148, y=w178) -> (x != y?=w151:bool)
                    n120 = Array Size(array=w209) -> (size(s)=w208:i32)
                    n121 = Bundle(w209, w205) -> (w126:cluster{timestamp[], dbl[]})  [unwired: 1 in]
                    n122 = Decrement(x=w208) -> (x-1=w207:i32)
                    n123 = Index Array(array=w209, index #2=w207) -> (element #1=w156:timestamp, element #2=w146:timestamp)  [unwired: 1 in]
                    n124 = case shown="真" w161 {
                      tunnel: [w234 w236] -> w145
                      tunnel: w137 -> [w234 w242]
                      tunnel: w132 -> [_ w235]
                      tunnel: w169 -> [w233 w241]
                      tunnel: w159 -> [_ w238]
                      tunnel: [w233 w237] -> w142
                      tunnel: w147 -> [_ w240]
                      tunnel: w146 -> [_ w239]
                      frame False {
                        # "不插入"
                      }
                      frame True {
                        # "尾插入 两点"
                        n125 = Insert Into Array(array=w241, new element #1=w239, new element #2=w238) -> (w237:timestamp[])  [unwired: 1 in]
                        n126 = Insert Into Array(array=w242, new element #1=w240, new element #2=w235) -> (w236:dbl[])  [unwired: 1 in]
                      }
                    }
                    n127 = case shown="真" w151 {
                      tunnel: [w251 w255] -> w188
                      tunnel: w138 -> [w251 w259]
                      tunnel: w178 -> [_ w252]
                      tunnel: w159 -> [_ w253]
                      tunnel: w187 -> [w250 w258]
                      tunnel: [w250 w254] -> w144
                      tunnel: w148 -> [_ w257]
                      tunnel: w146 -> [_ w256]
                      frame False {
                        # "不插入"
                      }
                      frame True {
                        # "尾插入 两点"
                        n128 = Insert Into Array(array=w259, new element #1=w257, new element #2=w252) -> (w255:dbl[])  [unwired: 1 in]
                        n129 = Insert Into Array(array=w258, new element #1=w256, new element #2=w253) -> (w254:timestamp[])  [unwired: 1 in]
                      }
                    }
                    n130 = Index Array(array=w142) -> (element=w141:timestamp)  [unwired: 1 in]
                    n131 = Index Array(array=w144) -> (element=w143:timestamp)  [unwired: 1 in]
                    n132 = Less? "过时？"(x=w141, y=w156) -> (x < y?=w168:bool)
                    n133 = Less? "过时？"(x=w143, y=w156) -> (x < y?=w186:bool)
                    n134 = Or(x=w136, y=w186) -> (x .or. y?=w140:bool)
                    n135 = Or(x=w135, y=w168) -> (x .or. y?=w139:bool)
                    n136 = case shown="真" w139 {
                      tunnel: w145 -> [w227 w231]
                      tunnel: w142 -> [w226 w230]
                      tunnel: 0 ("索引") -> [_ w232]
                      tunnel: [w227 w229] -> w134
                      tunnel: [w226 w228] -> w173
                      frame False {
                      }
                      frame True {
                        # "头删除"
                        n137 = Delete From Array(array=w231, index=w232) -> (array with subset deleted=w229:dbl[])  [unwired: 1 in, 1 out]
                        n138 = Delete From Array(array=w230, index=w232) -> (array with subset deleted=w228:timestamp[])  [unwired: 1 in, 1 out]
                      }
                    }
                    n139 = case shown="真" w140 {
                      tunnel: w188 -> [w244 w249]
                      tunnel: w144 -> [w243 w247]
                      tunnel: 0 ("索引") -> [_ w248]
                      tunnel: [w244 w246] -> w133
                      tunnel: [w243 w245] -> w157
                      frame False {
                      }
                      frame True {
                        # "头删除"
                        n140 = Delete From Array(array=w249, index=w248) -> (array with subset deleted=w246:dbl[])  [unwired: 1 in, 1 out]
                        n141 = Delete From Array(array=w247, index=w248) -> (array with subset deleted=w245:timestamp[])  [unwired: 1 in, 1 out]
                      }
                    }
                    n142 = Array Size(array=w133) -> (size(s)=w190:i32)
                    n143 = Array Size(array=w134) -> (size(s)=w172:i32)
                    n144 = Array Max & Min "最小限值2"(array=w134) -> (min value=w128:dbl)  [unwired: 3 out]
                    n145 = Array Max & Min "最大限值1"(array=w133) -> (max value=w131:dbl, min value=w130:dbl)  [unwired: 2 out]
                    n146 = Decrement(x=w190) -> (x-1=w191:i32)
                    n147 = Decrement(x=w172) -> (x-1=w171:i32)
                    n148 = Index Array(array=w133, index #2=w191) -> (element #1=w155:dbl, element #2=w154:dbl)  [unwired: 1 in]
                    n149 = Index Array(array=w134, index #2=w171) -> (element #1=w174:dbl, element #2=w175:dbl)  [unwired: 1 in]
                    n150 = Array Max & Min(array=w205) -> (max value=w196:dbl, min value=w195:dbl)  [unwired: 2 out]
                    n151 = Build Array (concatenate)(w155, w133, w154) -> (w153:dbl[])
                    n152 = Build Array (concatenate)(w156, w157, w146) -> (w152:timestamp[])
                    n153 = Build Array (concatenate)(w174, w134, w175) -> (w177:dbl[])
                    n154 = Build Array (concatenate)(w156, w173, w146) -> (w176:timestamp[])
                    n155 = control-ref of="XY图"() -> (w125:refnum<vi>)
                    n156 = Not Equal?(x=inf, y=w178) -> (x != y?=w193:bool)
                    n157 = case shown="真" w193 {
                      tunnel: w196 -> [w261 w267]
                      tunnel: [w261 w266] -> w129
                      tunnel: w130 -> [_ w265]
                      tunnel: w195 -> [w260 w264]
                      tunnel: [w260 w263] -> w194
                      tunnel: w131 -> [_ w262]
                      frame False {
                        # "报警限值 Inf 无效"
                      }
                      frame True {
                        # "报警限值有效"
                        n158 = Max & Min(x=w267, y=w262) -> (max(x,y)=w266:dbl)  [unwired: 1 out]
                        n159 = Max & Min(x=w264, y=w265) -> (min(x,y)=w263:dbl)  [unwired: 1 out]
                      }
                    }
                    n160 = Bundle(w152, w153) -> (w212:cluster{timestamp[], dbl[]})  [unwired: 1 in]
                    n161 = Bundle(w176, w177) -> (w158:cluster{timestamp[], dbl[]})  [unwired: 1 in]
                    n162 = Greater?(x=w129, y=w128) -> (0:w127:bool)
                    n163 = Subtract(x=w129, y=w194) -> (x-y=w204:dbl)
                    n164 = Multiply(x=w204, y=0.1) -> (x*y=w201:dbl)
                    n165 = Subtract(x=w156, y=w225) -> (x-y=w223:dbl)
                    n166 = Subtract(x=w146, y=w225) -> (x-y=w224:dbl)
                    n167 = Add(x=w129, y=w201) -> (x+y=w202:dbl)
                    n168 = Subtract(x=w194, y=w201) -> (x-y=w197:dbl)
                    n169 = property on="属性节点" class="XY图 (严格)"(reference=w125, "Active Plot"=w211, "Plot.Visible?"=w127) -> (error out=w206:errorcluster)  [unwired: 1 in, 1 out]
                    n170 = Less Or Equal To 0?(x=w197) -> (x <= 0?=w200:bool)
                    n171 = Select(t=0.0, s=w200, f=w197) -> (s? t:f=w198:dbl)
                    n172 = property on="属性节点" class="XYGraph (严格)"(reference=w125, error in=w206, "XScale.Maximum"=w224, "XScale.Minimum"=w223, "YScale.Maximum"=w202, "YScale.Minimum"=w198) -> ()  [unwired: 2 out]
                    n173 = in-place-match #2(w126) -> (w117:cluster{timestamp[], dbl[]})
                    n174 = in-place-match #3(w212) -> (w119:cluster{timestamp[], dbl[]})
                    n175 = in-place-match #4(w158) -> (w118:cluster{timestamp[], dbl[]})
                  }
                  n176 = in-place-array #1(w117, w119, w118) -> (w109:cluster{timestamp[], dbl[]}[])  [unwired: 3 out]
                }
                n177 = property on="坐标映射信号" class="Bool (严格)"("Val(Sgnl)"=w107) -> ()  [unwired: 2 in, 2 out]
                n178 = local write "XY图"(w109) -> ()
              }
            }
            n179 = Greater?(x=w50, y=w49) -> (0:w57:bool)
            n180 = case shown="真" w57 {
              tunnel: w50 -> [w102 w105]
              tunnel: w49 -> [_ w104]
              tunnel: [w102 w103] -> w52
              frame False {
                # "uSv/h"
              }
              frame True {
                # "mSv/h"
                n181 = Divide(x=w105, y=w104) -> (x/y=w103:dbl)
              }
            }
            n182 = Select(t=" m" ("F-格式字符串"), s=w57, f=" μ" ("F-格式字符串")) -> (s? t:f=w53:string)
            n183 = Number To Fractional String(number=w52, precision (6)=i16 2 ("精度(6)")) -> (F-format string=w56:string)  [unwired: 2 in]
            n184 = Concatenate Strings(w56, w53) -> (w51:string)
            n185 = Concatenate Strings("二级限值(Sv)：" ("字符串"), w51) -> (→"累积剂量":string)
          }
          event "坐标映射信号": Value Change {
            n186 = event-data() -> ()  [unwired: 1 in, 6 out]
            n187 = stacked-sequence {
              tunnel: [w323] -> w316
              frame #0 {
                n188 = Get Date/Time In Seconds() -> (seconds since 1Jan1904=w323:timestamp)
              }
            }
            n189 = Unbundle(w311) -> (w319:timestamp[], w318:dbl[])
            n190 = property on="数值" class="Str"() -> ("Visible"=w313:bool)  [unwired: 2 in, 2 out]
            n191 = Empty Array?(array=w318) -> (empty?=w317:bool)
            n192 = Not(x=w317) -> (.not. x?=w312:bool)
            n193 = And(x=w312, y=w313) -> (x .and. y?=w314:bool)
            n194 = case shown="真" w314 {
              tunnel: w319 -> [_ w345]
              tunnel: w318 -> [_ w344]
              tunnel: w316 -> [w324 w338]
              tunnel: [w324 w338] -> w315
              frame False {
                # "空数组，或悬浮数值不可见"
              }
              frame True {
                w355 = 1000.0 ("y")
                # "非空数组，且悬数值可见"
                n195 = control-ref of="XY图"() -> (w336:refnum<vi>)
                n196 = invoke on="调用节点" class="XY图 (严格)" method="Map Coords To XY"(reference=w336, "Coords"="鼠标坐标") -> ("XY"=w357:cluster{"X":dbl, "Y":dbl})  [unwired: 5 in, 6 out]
                n197 = Unbundle By Name("鼠标坐标") -> ("Horizontal"=w328:i32, "Vertical"=w327:i32)
                n198 = property on="数值" class="Str"() -> (error out=w340:errorcluster, "Bounds"=w339:T8)  [unwired: 2 in, 1 out]
                n199 = Unbundle By Name(w339) -> ("Width"=w330:u32, "Height"=w329:u32)
                n200 = Unbundle By Name(w357) -> ("X"=w350:dbl)
                n201 = Subtract(x=w345, y=timestamp(0 s since 1904-01-01)) -> (x-y=w348:dbl[])
                n202 = Divide(x=w330, y=u32 2) -> (x/y=w332:dbl)
                n203 = call "快速逼近索引法.vi"("数值"=w350, "数组"=w348) -> ("最近索引"=w347:i32)  [unwired: 9 in]
                n204 = Subtract(x=w328, y=w332) -> (x-y=w326:dbl)
                n205 = Index Array(array=w344, index=w347) -> (element=w346:dbl)
                n206 = Subtract(x=w327, y=w329) -> (x-y=w333:u32)
                n207 = Subtract(x=w333, y=u32 10) -> (x-y=w325:u32)
                n208 = Greater Or Equal?(x=w346, y=w355) -> (x >= y?=w356:bool)
                n209 = case shown="假" w356 {
                  tunnel: w346 -> [w359 w363]
                  tunnel: w355 -> [_ w362]
                  tunnel: [w359 w361] -> w353
                  tunnel: [" μSv/h" " mSv/h"] -> w351
                  frame False {
                    # "mSv/h"
                  }
                  frame True {
                    # "uSv/h"
                    n210 = Divide(x=w363, y=w362) -> (x/y=w361:dbl)
                  }
                }
                n211 = Bundle By Name(cluster=T5 {"Left"=0, "Top"=0} ("位置"), "Left"=w326, "Top"=w325) -> (w342:T5)
                n212 = property on="数值" class="Str"(error in=w340, "Position"=w342) -> ()  [unwired: 1 in, 2 out]
                n213 = Number To Fractional String(number=w353, precision (6)=i16 2 ("精度(6)")) -> (F-format string=w352:string)  [unwired: 2 in]
                n214 = Concatenate Strings(w352, w351) -> (→"数值":string)
                n215 = Wait (ms)(milliseconds to wait=u32 30 ("等待时间（毫秒）")) -> ()  [unwired: 1 out]
              }
            }
            n216 = stacked-sequence {
              tunnel: w315 -> [w321]
              frame #0 {
                # "净处理时间为\n最少 3μs\n300点满数组 5~20ms"
                n217 = Get Date/Time In Seconds() -> (seconds since 1Jan1904=w322:timestamp)
                n218 = Subtract(x=w322, y=w321) -> (x-y=→"计算时间":dbl)
              }
            }
          }
          event "XY图": Mouse Enter {
            w364 = TRUE  # T
            n219 = event-data() -> ()  [unwired: 1 in, 4 out]
            n220 = property on="数值" class="Str"("Visible"=w364) -> ()  [unwired: 2 in, 2 out]
          }
          event "XY图": Mouse Leave {
            w366 = FALSE  # F
            n221 = event-data() -> ()  [unwired: 1 in, 4 out]
            n222 = property on="数值" class="Str"("Visible"=w366) -> ()  [unwired: 2 in, 2 out]
          }
          event "XY图": Mouse Move {
            n223 = event-data() -> ("Coords"=w368:T1)  [unwired: 1 in, 4 out]
            n224 = flat-sequence {
              tunnel: w368 -> [w370]
              frame #0 {
                n225 = local write "鼠标坐标"(w370) -> ()
              }
              frame #1 {
                n226 = property on="坐标映射信号" class="Bool (严格)"("Val(Sgnl)"=FALSE ("值(信号)")) -> ()  [unwired: 2 in, 2 out]
              }
            }
          }
          event "探头状态": Value Change {
            n227 = event-data() -> ("OldVal"=w375:T3, "NewVal"=w373:T3)  [unwired: 1 in, 4 out]
            n228 = Equal?(x=w375, y=w373) -> (x = y?=w374:bool)
            n229 = case shown="假" w374 {
              tunnel: w373 -> [w381 _]
              frame False {
                # "不相等，值改变"
                n230 = case shown="\"累积报警\"" w381 {
                  tunnel: [w405 w407 w410 w412 w413 w416] -> w377
                  tunnel: [u32 0 u32 8618883 w409 w411 w414 w415] -> w376
                  frame "正常", Default {
                    w405 = u32 14869218  # 正常
                  }
                  frame "离线" {
                    w407 = u32 14869218  # 离线
                  }
                  frame "一级报警" {
                    w409 = u32 1440533  # 文字
                    w410 = u32 16711680  # 一级背景
                  }
                  frame "二级报警" {
                    w411 = u32 1440533  # 文字
                    w412 = u32 16711680  # 二级背景
                  }
                  frame "未启用" {
                    w413 = u32 14869218  # 正常
                    w414 = u32 8816262  # 禁用
                  }
                  frame "累积报警" {
                    n231 = disable-structure shown="启用" {
                      disable-tunnel: [w418 w420] -> w416
                      disable-tunnel: [w417 u32 0] -> w415
                      frame Disabled {
                        w417 = u32 1440533  # 文字
                        w418 = u32 16711680  # 一级背景
                      }
                      frame Enabled {
                        w420 = u32 14869218  # 正常
                      }
                    }
                  }
                }
                n232 = control-ref of="单位"() -> (w393:refnum<vi>)
                n233 = control-ref of="探头信息"() -> (w394:refnum<vi>)
                n234 = control-ref of="限值1"() -> (w391:refnum<vi>)
                n235 = control-ref of="探头地址"() -> (w397:refnum<vi>)
                n236 = control-ref of="限值2"() -> (w392:refnum<vi>)
                n237 = control-ref of="探头状态"() -> (w395:refnum<vi>)
                n238 = control-ref of="测量值"() -> (w396:refnum<vi>)
                n239 = property on="属性节点" class="DigNum (严格)"(reference=w396, "NumText.TextColor"=w376) -> ("OwningPane"=w399:refnum<vi>)  [unwired: 1 in, 2 out]
                n240 = property on="属性节点" class="Enum (严格)"(reference=w397, "RingText.TextColor"=w376) -> ("OwningPane"=w398:refnum<vi>)  [unwired: 1 in, 2 out]
                n241 = property on="属性节点" class="Enum (严格)"(reference=w395, "RingText.TextColor"=w376) -> ("OwningPane"=w400:refnum<vi>)  [unwired: 1 in, 2 out]
                n242 = property on="属性节点" class="Enum (严格)"(reference=w393, "RingText.TextColor"=w376) -> ("OwningPane"=w402:refnum<vi>)  [unwired: 1 in, 2 out]
                n243 = property on="属性节点" class="Str"(reference=w394, "Text.TextColor"=w376) -> ("OwningPane"=w401:refnum<vi>)  [unwired: 1 in, 2 out]
                n244 = property on="属性节点" class="Str"(reference=w392, "Text.TextColor"=w376) -> ("OwningPane"=w403:refnum<vi>)  [unwired: 1 in, 2 out]
                n245 = property on="属性节点" class="Str"(reference=w391, "Text.TextColor"=w376) -> ("OwningPane"=w404:refnum<vi>)  [unwired: 1 in, 2 out]
                n246 = property on="累积剂量" class="Str"("Text.TextColor"=w376) -> ("OwningPane"=w379:refnum<vi>)  [unwired: 2 in, 2 out]
                n247 = control-ref of="窗格 7"() -> (w380:refnum<vi>)
                n248 = property class="Pane"(reference=w398, "PaneColor"=w377) -> ()  [unwired: 1 in, 2 out]
                n249 = property class="Pane"(reference=w399, "PaneColor"=w377) -> ()  [unwired: 1 in, 2 out]
                n250 = property class="Pane"(reference=w400, "PaneColor"=w377) -> ()  [unwired: 1 in, 2 out]
                n251 = property class="Pane"(reference=w401, "PaneColor"=w377) -> ()  [unwired: 1 in, 2 out]
                n252 = property class="Pane"(reference=w402, "PaneColor"=w377) -> ()  [unwired: 1 in, 2 out]
                n253 = property class="Pane"(reference=w403, "PaneColor"=w377) -> ()  [unwired: 1 in, 2 out]
                n254 = property class="Pane"(reference=w404, "PaneColor"=w377) -> ()  [unwired: 1 in, 2 out]
                n255 = property class="Pane"(reference=w380, "PaneColor"=w377) -> ()  [unwired: 1 in, 2 out]
                n256 = property class="Pane"(reference=w379, "PaneColor"=w377) -> ()  [unwired: 1 in, 2 out]
                n257 = Bundle("正常"=w377, "正常"=w377) -> (w383:cluster{"正常":u32, "正常":u32})  [unwired: 1 in]
                n258 = control-ref of="分隔栏 2"() -> (w390:refnum<vi>)
                n259 = control-ref of="分隔栏 3"() -> (w389:refnum<vi>)
                n260 = control-ref of="分隔栏 4"() -> (w388:refnum<vi>)
                n261 = control-ref of="分隔栏 5"() -> (w387:refnum<vi>)
                n262 = control-ref of="分隔栏 6"() -> (w386:refnum<vi>)
                n263 = control-ref of="分隔栏 7"() -> (w385:refnum<vi>)
                n264 = control-ref of="分隔栏 8"() -> (w384:refnum<vi>)
                n265 = control-ref of="分隔栏 9"() -> (w378:refnum<vi>)
                n266 = Build Array(w390, w389, w388, w387, w386, w385, w384, w378) -> (w382:refnum<vi>[])
                n267 = for {
                  tunnel: w383 -> [w422]
                  workers-P: _ -> [_]
                  tunnel: w382 -> [w421] mode=indexing
                  n268 = property on="属性节点" class="Splitter"(reference=w421, "Colors"=w422) -> ()  [unwired: 1 in, 2 out]
                }
              }
              frame True {
              }
            }
          }
        }
      }
    }
  }
